vi "TCP Read.vi"(8 "error in (no error)":errorcluster, 9 "timeout (ms)":i32=5000, 11 "connection ID":refnum<k5>) -> (0 "error out":errorcluster, 2 "data string":string, 3 "connection ID 2":refnum<k5>)   [LabVIEW 2015]
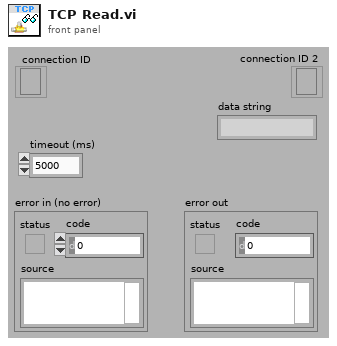
[diagram p1: front panel]
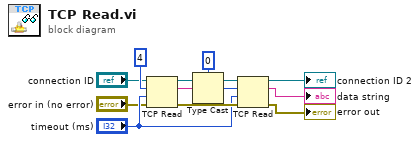
[diagram p0: block diagram]
diagram:
  n1 = TCP Read(connection ID="connection ID", bytes to read=4, error in (no error)="error in (no error)", 9:"timeout (ms)") -> (connection ID out=w10:refnum<k5>, data out=w7:string, error out=w9:errorcluster)  [unwired: 1 in]
  n2 = Type Cast(type=0, x=w7) -> (*(type *) &x=w2:i32)
  n3 = TCP Read(connection ID=w10, bytes to read=w2, error in (no error)=w9, 9:"timeout (ms)") -> (connection ID out=→"connection ID 2":refnum<k5>, data out=→"data string":string, error out=→"error out":errorcluster)  [unwired: 1 in]
